vi "Init and Rotate array Graf2.vi"(5 "Reset":bool, 7 "Stop read":bool, 9 "Array size":i32=30, 10 "PV":dbl[](array[numeric]), 11 "XY Graf in":cluster{"time stamp":timestamp[], "PV":dbl[]}[](array[cluster])) -> (3 "XY Graf out":cluster{"time stamp":timestamp[], "PV":dbl[]}[](array[cluster]))   [LabVIEW 2019, in "Userlib.lvlib"]
uses:
  Userlib.lvlib
panel:
  out "XY Graf out 2":cluster{"time stamp":timestamp[], "PV":dbl[]}[](array[cluster])
  in  "XY Graf in 2":cluster{"time stamp":timestamp[], "PV":dbl[]}[](array[cluster])
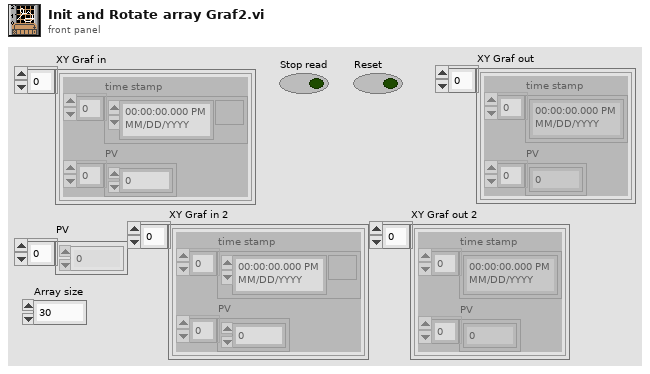
[diagram p1: front panel]
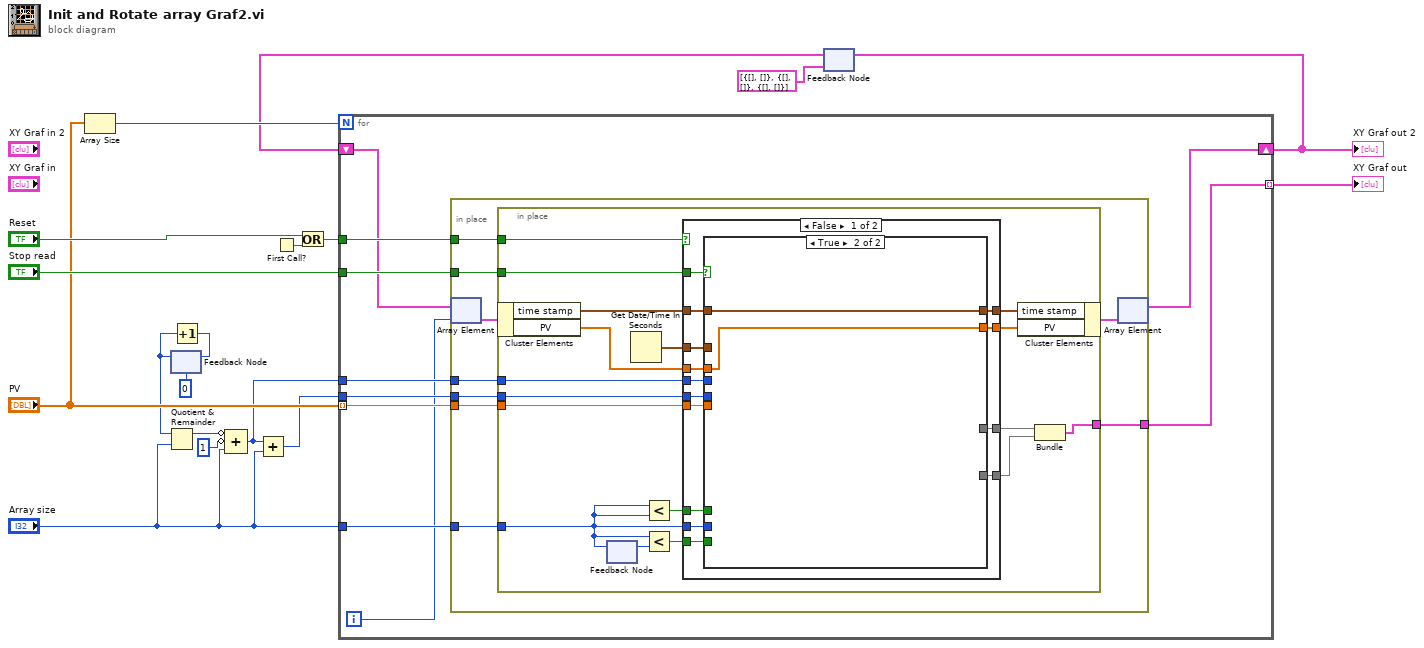
[diagram p0: block diagram]
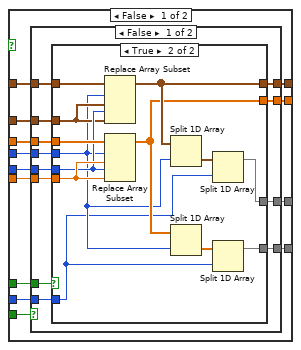
[diagram p2: hidden frame]
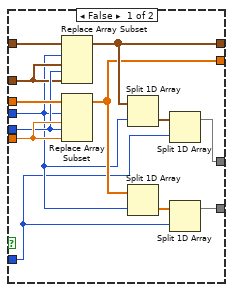
[diagram p3: hidden frame]
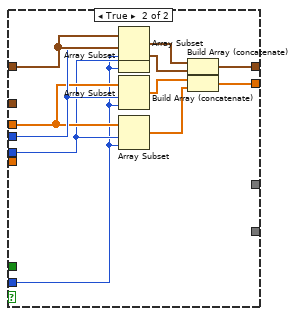
[diagram p4: hidden frame]
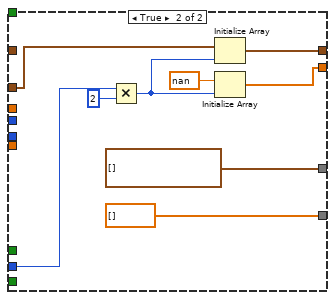
[diagram p5: hidden frame]
diagram:
  n1 = Array Size(array="PV") -> (size(s)=w15:i32)
  n2 = feedback #1(0 ("t")) -> (w11:i32)
  n3 = Quotient & Remainder(x=w11, y="Array size") -> (x-y*floor(x/y)=w10:i32)  [unwired: 1 out]
  n4 = Increment(x=w11) -> (x+1=w12:i32)
  n5 = feedback-in #1(w12) -> ()
  n6 = Compound Arithmetic op=ADD(invert w10, invert 1 ("value"), "Array size") -> (w7:i32)
  n7 = Add(x=w7, y="Array size") -> (x+y=w6:i32)
  n8 = First Call?() -> (First Call?: T/F=w4:bool)
  n9 = Or(x="Reset", y=w4) -> (x .or. y?=w5:bool)
  n10 = feedback #2(cluster{"time stamp":timestamp[], "PV":dbl[]}[] [{"time stamp"=[], "PV"=[]}, {"time stamp"=[], "PV"=[]}, {"time stamp"=[], "PV"=[]}] ("XY Graf out")) -> (w2:cluster{"time stamp":timestamp[], "PV":dbl[]}[])
  n11 = for {
    N: w15 -> [_]
    tunnel: "Stop read" -> [w28]
    tunnel: w5 -> [w27]
    tunnel: "PV" -> [w26] mode=indexing
    tunnel: "Array size" -> [w25]
    shift-right: [w20] -> w3
    shift-left: w2 -> [w22]
    tunnel: w7 -> [w24]
    tunnel: w6 -> [w23]
    tunnel: [w19] -> w16 mode=indexing
    i -> [w21]
    n12 = in-place {
      in-place-border: w28 -> [w37]
      in-place-border: w27 -> [w36]
      in-place-border: w26 -> [w35]
      in-place-border: w25 -> [w34]
      in-place-border: w24 -> [w33]
      in-place-border: w23 -> [w32]
      in-place-border: [w29] -> w19
      n13 = in-place-array #3(w22, w21) -> (w31:cluster{"time stamp":timestamp[], "PV":dbl[]})
      n14 = in-place {
        in-place-border: w37 -> [w54]
        in-place-border: w36 -> [w51]
        in-place-border: w35 -> [w53]
        in-place-border: w34 -> [w38]
        in-place-border: w33 -> [w45]
        in-place-border: w32 -> [w44]
        in-place-border: [w39] -> w29
        n15 = in-place-cluster #4(w31) -> ("time stamp"=w47:timestamp[], "PV"=w43:dbl[])
        n16 = feedback #5() -> (w50:i32)  [unwired: 1 in]
        n17 = feedback-in #5(w38) -> ()
        n18 = Get Date/Time In Seconds() -> (seconds since 1Jan1904=w52:timestamp)
        n19 = Less?(x=w38, y=w38) -> (x < y?=w48:bool)
        n20 = Less?(x=w38, y=w50) -> (x < y?=w49:bool)
        n21 = case shown="False" w51 {
          tunnel: w54 -> [w62 _]
          tunnel: w53 -> [w68 _]
          tunnel: w52 -> [w67 w139]
          tunnel: [w66 timestamp[] [] ("time stamp")] -> w41
          tunnel: [w65 dbl[] [] ("PV")] -> w40
          tunnel: w49 -> [w61 _]
          tunnel: w38 -> [w64 w138]
          tunnel: w48 -> [w63 _]
          tunnel: w47 -> [w60 _]
          tunnel: [w59 w134] -> w46
          tunnel: w45 -> [w58 _]
          tunnel: w44 -> [w57 _]
          tunnel: w43 -> [w56 _]
          tunnel: [w55 w135] -> w42
          frame False {
            n22 = case shown="True" w62 {
              tunnel: w61 -> [w77 _]
              tunnel: w68 -> [w81 _]
              tunnel: w67 -> [w80 _]
              tunnel: [w79 _] -> w66
              tunnel: [w78 _] -> w65
              tunnel: w64 -> [w75 _]
              tunnel: w63 -> [w76 _]
              tunnel: w60 -> [w74 w132]
              tunnel: [w73 w132] -> w59
              tunnel: w58 -> [w72 _]
              tunnel: w57 -> [w71 _]
              tunnel: w56 -> [w70 w131]
              tunnel: [w69 w131] -> w55
              frame False {
                n23 = case shown="False" w77 {
                  tunnel: w81 -> [w93 _]
                  tunnel: w80 -> [w92 _]
                  tunnel: [w91 _] -> w78
                  tunnel: [w90 _] -> w79
                  tunnel: w76 -> [w89 _]
                  tunnel: w75 -> [w82 w126]
                  tunnel: w74 -> [w88 w130]
                  tunnel: [w87 w123] -> w73
                  tunnel: w72 -> [w86 w129]
                  tunnel: w71 -> [w85 w127]
                  tunnel: w70 -> [w84 w128]
                  tunnel: [w83 w120] -> w69
                  frame False {
                    n24 = case shown="True" w89 {
                      tunnel: w92 -> [w102 w115]
                      tunnel: w93 -> [w104 w117]
                      tunnel: [w99 w112] -> w90
                      tunnel: [w95 w108] -> w91
                      tunnel: w88 -> [w106 w119]
                      tunnel: [w101 w114] -> w87
                      tunnel: w86 -> [w97 w110]
                      tunnel: w85 -> [w103 w116]
                      tunnel: w84 -> [w105 w118]
                      tunnel: [w98 w111] -> w83
                      tunnel: w82 -> [w94 w107]
                      frame False {
                        n25 = Replace Array Subset(array=w106, new element #1=w102, index #1=w97, new element #2=w102, index #2=w103) -> (w101:timestamp[])
                        n26 = Replace Array Subset(array=w105, new element #1=w104, index #1=w97, new element #2=w104, index #2=w103) -> (w98:dbl[])
                        n27 = Split 1D Array(array=w101, index=w97) -> (second subarray=w100:timestamp[])  [unwired: 1 out]
                        n28 = Split 1D Array(array=w98, index=w97) -> (second subarray=w96:dbl[])  [unwired: 1 out]
                        n29 = Split 1D Array(array=w100, index=w94) -> (first subarray=w99:timestamp[])  [unwired: 1 out]
                        n30 = Split 1D Array(array=w96, index=w94) -> (first subarray=w95:dbl[])  [unwired: 1 out]
                      }
                      frame True {
                        n31 = Replace Array Subset(array=w119, new element #1=w115, index #1=w110, new element #2=w115, index #2=w116) -> (w114:timestamp[])
                        n32 = Replace Array Subset(array=w118, new element #1=w117, index #1=w110, new element #2=w117, index #2=w116) -> (w111:dbl[])
                        n33 = Split 1D Array(array=w114, index=w110) -> (second subarray=w113:timestamp[])  [unwired: 1 out]
                        n34 = Split 1D Array(array=w111, index=w110) -> (second subarray=w109:dbl[])  [unwired: 1 out]
                        n35 = Split 1D Array(array=w113, index=w107) -> (first subarray=w112:timestamp[])  [unwired: 1 out]
                        n36 = Split 1D Array(array=w109, index=w107) -> (first subarray=w108:dbl[])  [unwired: 1 out]
                      }
                    }
                  }
                  frame True {
                    n37 = Array Subset(array=w130, index=w129, length=w126) -> (w125:timestamp[])
                    n38 = Array Subset(array=w130, index=w127, length=w126) -> (w124:timestamp[])
                    n39 = Array Subset(array=w128, index=w129, length=w126) -> (w122:dbl[])
                    n40 = Array Subset(array=w128, index=w127, length=w126) -> (w121:dbl[])
                    n41 = Build Array (concatenate)(w125, w124) -> (w123:timestamp[])
                    n42 = Build Array (concatenate)(w122, w121) -> (w120:dbl[])
                  }
                }
              }
              frame True {
              }
            }
          }
          frame True {
            n43 = Multiply(x=w138, y=2) -> (x*y=w133:i32)
            n44 = Initialize Array(w139, w133) -> (w134:timestamp[])
            n45 = Initialize Array(nan ("PV"), w133) -> (w135:dbl[])
          }
        }
        n46 = in-place-cluster #4("time stamp"=w46, "PV"=w42) -> (w30:cluster{"time stamp":timestamp[], "PV":dbl[]})
        n47 = Bundle("time stamp"=w41, "PV"=w40) -> (w39:cluster{"time stamp":timestamp[], "PV":dbl[]})  [unwired: 1 in]
      }
      n48 = in-place-array #3(w30) -> (w20:cluster{"time stamp":timestamp[], "PV":dbl[]}[])  [unwired: 1 out]
    }
  }
  "XY Graf out" <- w16
  "XY Graf out 2" <- w3
  n49 = feedback-in #2(w3) -> ()
